vi "Create.vi"(7 "Group":string="Default", 8 "error in (no error)":errorcluster, 10 "Tag":string, 11 "Blackboard":refnum<class "Blackboard.lvclass">) -> (0 "error out":errorcluster, 2 "Blackboard_Boolean.lvclass":refnum<class "Blackboard_String.lvclass">, 3 "Blackboard Out":refnum<class "Blackboard.lvclass">)   [LabVIEW 2021, in "Blackboard_String.lvclass"]
uses:
  Blackboard_String.lvclass
  C:/Program Files (x86)/National Instruments/LabVIEW 2021/vi.lib/TSA/Abstract Data Classes/Abs_Types/Type/Abs_Type.lvclass
  Blackboard.lvclass
  Blackboard_String.lvclass/Blackboard_String.ctl
  <vilib>/TSA/Abstract Data Classes/Abs_Types/Type/Abs_Type.lvclass/Abs_Type.ctl
  Properties/Write Blackboard.vi
  Properties/Write Group.vi
  Properties/Write Write.vi
  Properties/Read Blackboard.vi
  <vilib>/TSA/Abstract Data Classes/Abs_Types/Type/Abs_Type.lvclass
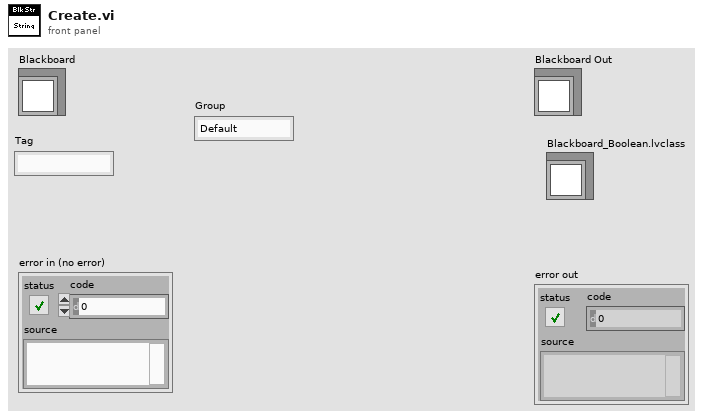
[diagram p1: front panel]
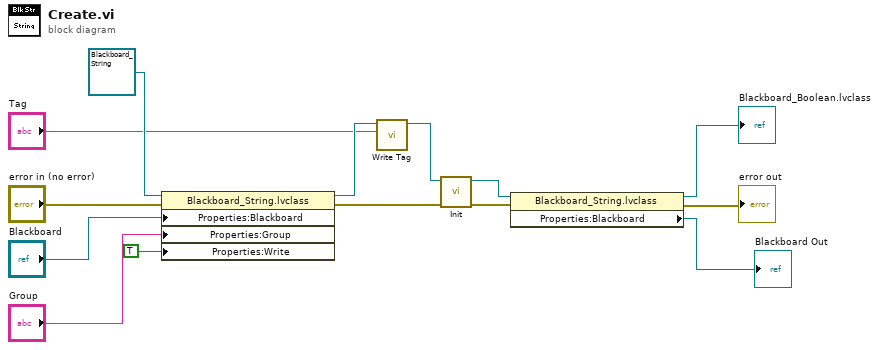
[diagram p0: block diagram]
diagram:
  n1 = property class="Blackboard_String.lvclass"(reference=refnum<class "Blackboard_String.lvclass"> refnum ("Blackboard_Boolean.lvclass"), error in="error in (no error)", "Properties:Blackboard"="Blackboard", "Properties:Group"="Group", "Properties:Write"=TRUE ("Write")) -> (reference out=w9:refnum<class "Blackboard_String.lvclass">, error out=w6:errorcluster)
  n2 = call <vilib>:"Write Tag.vi"("Tag"="Tag", "Abs_Type in"=w9) -> ("Abs_Type out"=w8:refnum<class "Blackboard_String.lvclass">)  [unwired: 9 in]
  n3 = call-dynamic "Init.vi"("error in (no error)"=w6, "Data in"=w8) -> ("error out"=w5:errorcluster, "Data out"=w4:refnum<class "Blackboard_String.lvclass">)  [unwired: 8 in]
  n4 = property class="Blackboard_String.lvclass"(reference=w4, error in=w5) -> (reference out=→"Blackboard_Boolean.lvclass":refnum<class "Blackboard_String.lvclass">, error out=→"error out":errorcluster, "Properties:Blackboard"=→"Blackboard Out":refnum<class "Blackboard.lvclass">)
